vi "Initialize.vi"(6 "Actor Name":string, 7 "Host Name":string, 8 "error in (no error)":errorcluster, 11 "Message Broker":refnum<class "Message Broker Interface Ref.lvclass">) -> (0 "error out":errorcluster, 3 "Terminal Timeout out":refnum<class "Terminal Timeout.lvclass">)   [LabVIEW 2016, in "CLD Exam - ATM.lvlib" / "Terminal Timeout.lvclass"]
uses:
  Terminal Timeout.lvclass
  Mediator/Classes/Message Broker Interface Ref/Message Broker Interface Ref.lvclass
  D:/Repos/Stream/software/Mediator/Classes/Message Broker Interface/Message Broker Interface.lvclass
  Terminal Timeout.lvclass/Terminal Timeout.ctl
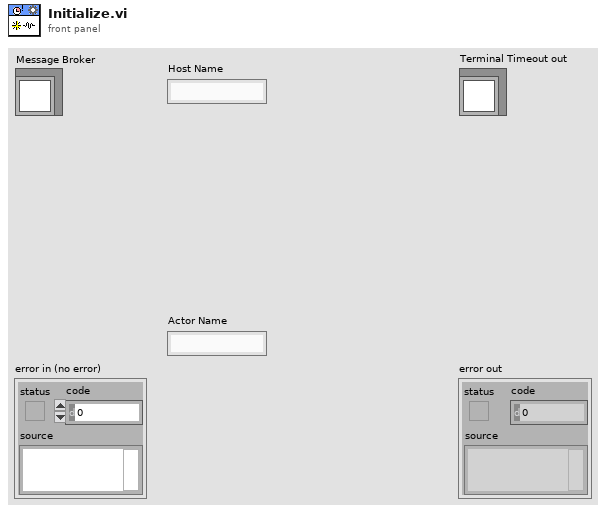
[diagram p1: front panel]
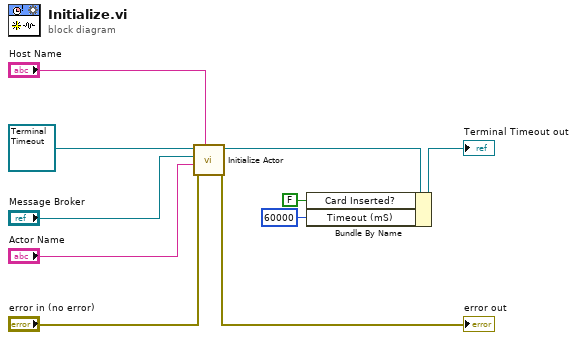
[diagram p0: block diagram]
diagram:
  n1 = call-dynamic "Initialize Actor.vi"("Host Name"="Host Name", "error in (no error)"="error in (no error)", "Actor Name"="Actor Name", "Message Broker Interface"="Message Broker", "Terminal Timeout in"=refnum<class "Terminal Timeout.lvclass"> refnum) -> ("error out"=→"error out":errorcluster, "Terminal Timeout out"=w4:refnum<class "Terminal Timeout.lvclass">)  [unwired: 5 in]
  n2 = Bundle By Name(cluster=w4, "Card Inserted?"=FALSE ("Data.Card Inserted?"), "Timeout (mS)"=60000 ("Data.Timeout (mS)")) -> (→"Terminal Timeout out":refnum<class "Terminal Timeout.lvclass">)
